vi "Read Water Level Actor.vi"(11 "硬件蒸发冷却器":refnum<class "HW Evaporative Cooler.lvclass">) -> (2 "水位":refnum<class "Water Level.lvclass">)   [LabVIEW 2015, in "HW Evaporative Cooler.lvclass"]
uses:
  HW Evaporative Cooler.lvclass
  Water Level/Water Level.lvclass
  HW Water Level.lvclass/HW Water Level.lvclass
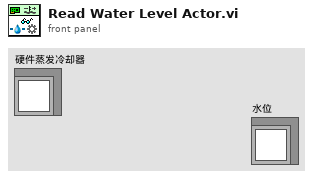
[diagram p1: front panel]
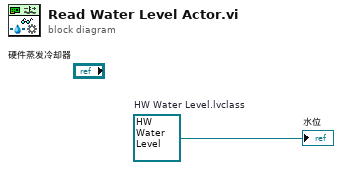
[diagram p0: block diagram]
diagram:
  w1 = refnum<class "HW Water Level.lvclass"> refnum  # HW Water Level.lvclass
  "水位" <- w1
